vi "enc2theta.vi"(8 "Enc 2":i32, 9 "Enc 1":i32, 10 "Enc 2 offset":i32, 11 "Enc 1 offset":i32) -> (2 "th":dbl[](array[numeric]))   [LabVIEW 2018]
uses:
  <vilib>/imath/engines/lvmath2/RunTimeEngine/IndexReplace/NIMS V(S)=S.vi
  <instcachedir>/0/NIMS V(S)=S_420DA4522869420292A92FA3CC108C4E.lvgen/NIMS V(S)=S_420DA4522869420292A92FA3CC108C4E_000.vi
  <vilib>/imathl/engines/lvmath/Functions/Error Handling/Create Error.vi
  <vilib>/imath/engines/lvmath2/RunTimeEngine/NodeEndStatement/NIMS_NodeEndStatement_Output.vi
  <instcachedir>/0/NIMS_NodeEndStatement_Output_53EC0D466D134D7ABD903AC30B43404B.lvgen/NIMS_NodeEndStatement_Output_53EC0D466D134D7ABD903AC30B43404B_005.vi
  <vilib>/imath/engines/lvmath2/RunTimeEngine/ErrorHandling/NIMS_Finalize Error.vi
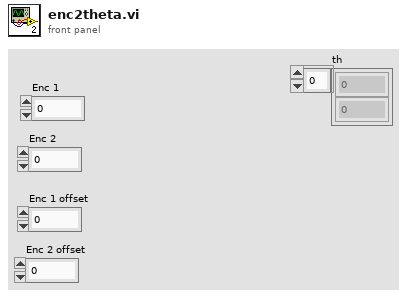
[diagram p1: front panel]
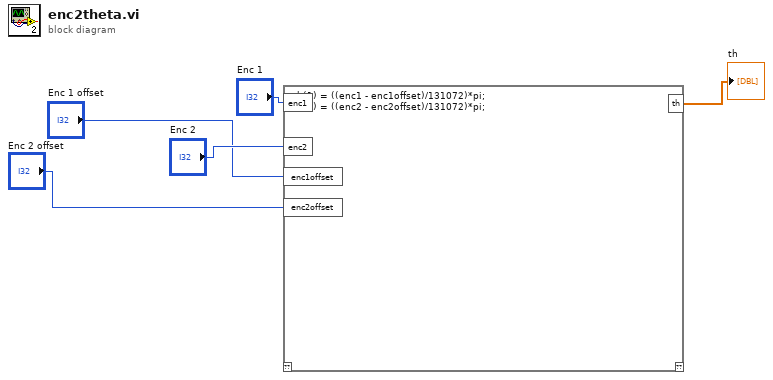
[diagram p0: block diagram]
diagram:
  n1 = mathscript code="th(1) = ((enc1 - enc1offset)/131072)*pi;\nth(2) = ((enc2 - enc2offset)/131072)*pi;"("enc1"="Enc 1", "enc2"="Enc 2", "enc1offset"="Enc 1 offset", "enc2offset"="Enc 2 offset") -> ("th"=→"th":dbl[])  [unwired: 1 in, 1 out]
